vi "RFSG List Mode Test Signal Generation for 5668 with calibrated Signal.vi"(0 "Resource Name":refnum<k15>="RFSG" caption="resource name", 5 "Start Frequency":dbl=3850000000.0 format="%#_6p", 7 "End Frequency":dbl=4800000000.0 format="%#_6p", 11 "error in (no error)":errorcluster) -> (4 "# Tones":i32, 15 "error out":errorcluster)   [LabVIEW 2017]
doc: "Demonstrates how to create a Configuration List for sweeping frequency and/or power."
uses:
  <instrlib>/niRFSG/niRFSG.llb/niRFSG Ref Clock Sources.ctl
  <instrlib>/niRFSG/niRFSG.llb/niRFSG Configuration List Properties.ctl
  <vilib>/Analysis/1siggen.llb/Ramp Pattern by Delta.vi
  <vilib>/Analysis/NI_AALBase.lvlib
panel:
  in  "delta":dbl=50000000.0 format="%#_6p"
  out "Ramp Pattern":dbl[](array[numeric]) format="%#_6p"
  in  "Power Level (dBm)":dbl format="%_3f"
  in  "Timer:Interval":dbl
  in  "List Trigger Source":string(combo)="PXI_Trig1"
  out "Current Frequency (Hz)":dbl format="%#.3p"
  in  "Frequency Settling (ppm)":dbl=1.0 format="%#.6f"
  in  "Stop":bool
  in  "Reference Clock Source":T1="OnboardClock"
  # "Overview: Demonstrates how to create a Configuration List for sweeping frequency and/or power.\nRequirements: NI-RFSG\nInstructions:\n1. Change the Resource Name to your device.\n2. Run the VI.\n3. Click Stop to stop the VI."
  # "You can set the Start Frequency and End Frequency parameters to the same value to keep the Frequency or Power Level constant."
  # "In order to configure new settings, you must stop the example using \nthe Stop button and then run the VI with the new settings."
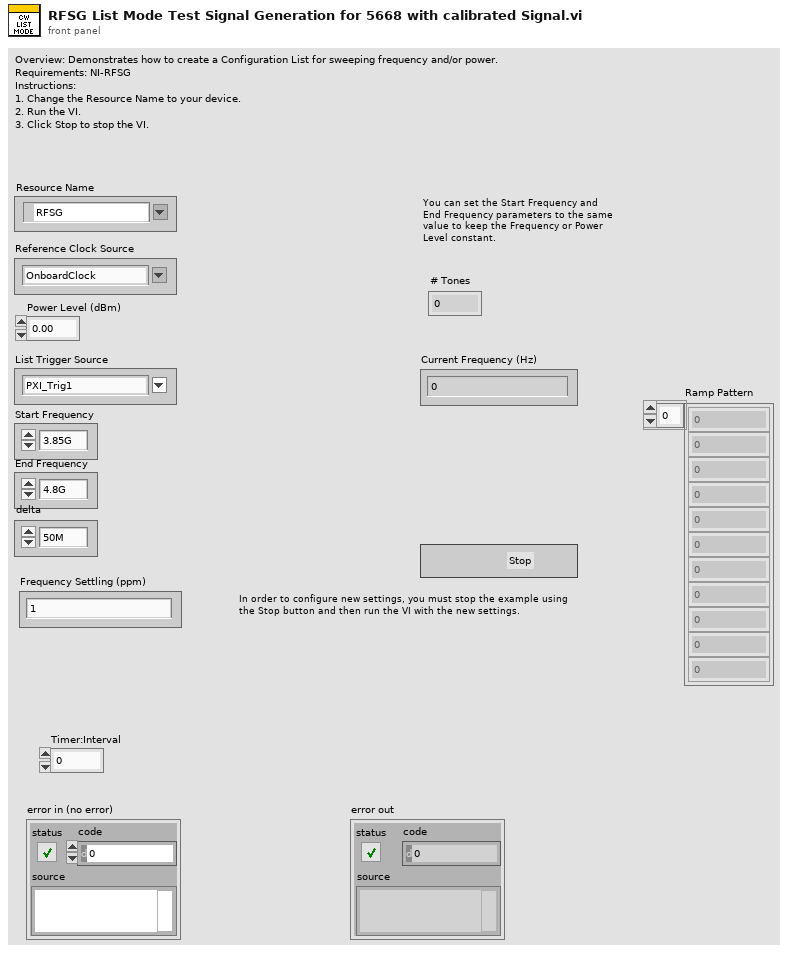
[diagram p1: front panel]
types:
  T1 = typedef "niRFSG Ref Clock Sources.ctl" = string
  T2 = typedef "niRFSG Configuration List Properties.ctl" = u32
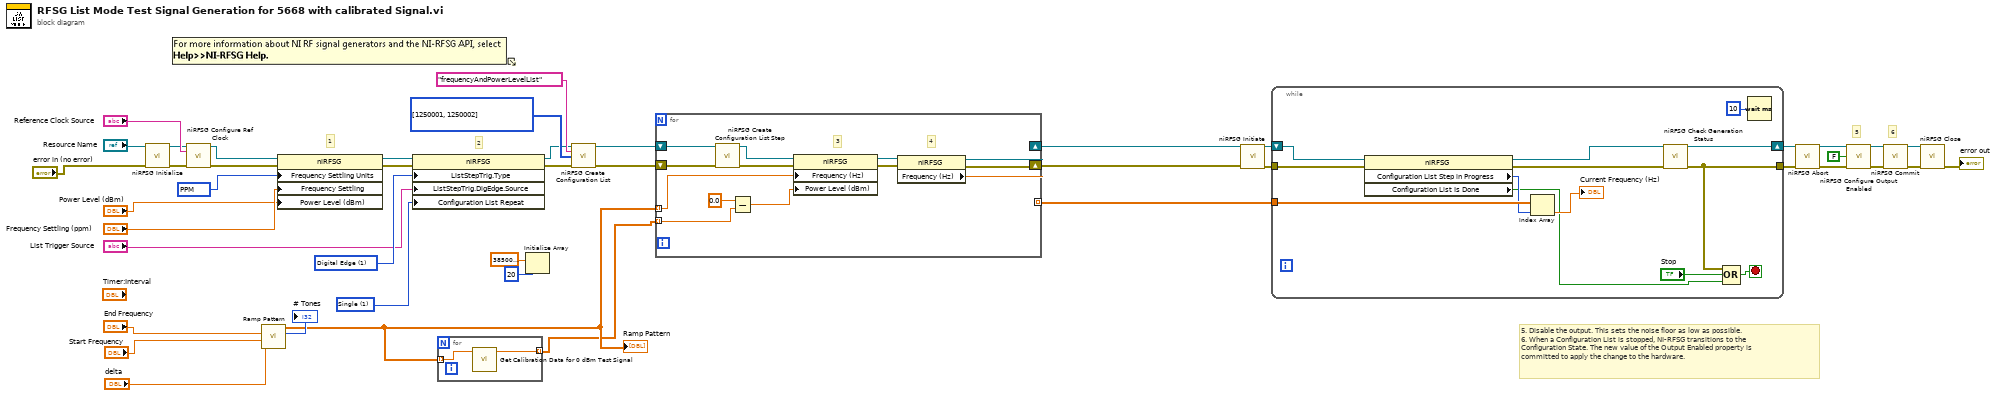
[diagram p0: block diagram]
diagram:
  w9 = 1 items=["Continuous", "Single"] ("Configuration List:Configuration List Repeat")
  w32 = T2[] [1250001, 1250002] items=["ALC Control"=1150195, "Amp Path"=1150185, "Amplitude Settling (dB)"=1150137, "Attenuator Setting (dB)"=1150173, "Automatic Power Search"=1150196, "Frequency (Hz)"=1250001, "Frequency Settling"=1150083, "IQ Out Port Carrier Frequency"=1150145, "IQ Out Port Common Mode Offset"=1150148, "IQ Out Port Level"=1150147, "IQ Out Port Offset"=1150149, "Output Enabled"=1250004, "Phase Offset (Degrees)"=1150024, "Power Level (dBm)"=1250002, "Pulse Modulation Enabled"=1250051, "Timer Event Interval (s)"=1150100, "Upconverter Center Frequency (Hz)"=1154098] ("configuration list properties")
  w39 = 1 items=["None", "Digital Edge", "Software"] ("Triggers:Configuration List Step:Type")
  w44 = 12002 items=["Seconds After Lock"=12000, "Seconds After I/O"=12001, "PPM"=12002] ("RF:Frequency Settling Units")
  # "6"
  # "2"
  # "5. Disable the output. This sets the noise floor as low as possible.\n6. When a Configuration List is stopped, NI-RFSG transitions to the Configuration State. The new value of the Output Enabled property is committed to apply the change to the hardware."
  # "5"
  # "1"
  n1 = call <instrlib>:"niRFSG Initialize.vi"("resource name"="Resource Name", "error in"="error in (no error)") -> ("instrument handle"=w22:refnum<k15>, "error out"=w21:errorcluster)  [unwired: 2 in, 10 out]
  n2 = call <instrlib>:"niRFSG Configure Ref Clock.vi"("instrument handle"=w22, "ref clock source"="Reference Clock Source", "error in"=w21) -> ("instrument handle out"=w11:refnum<k15>, "error out"=w26:errorcluster)  [unwired: 1 in, 10 out]
  n3 = call-poly <vilib>:"Ramp Pattern.vi"("start"="Start Frequency", "end"="End Frequency", "delta"="delta") -> ("samples"=→"# Tones":i32, "Ramp Pattern"=w2:dbl[])  [unwired: 6 in, 1 out]
  "Ramp Pattern" <- w2
  n4 = property class="niRFSG"(reference=w11, error in=w26, "Frequency Settling Units"=w44, "Frequency Settling"="Frequency Settling (ppm)", "Power Level (dBm)"="Power Level (dBm)") -> (reference out=w36:refnum<k15>, error out=w37:errorcluster)
  n5 = property class="niRFSG"(reference=w36, error in=w37, "ListStepTrig.Type"=w39, "ListStepTrig.DigEdge.Source"="List Trigger Source", "Configuration List Repeat"=w9) -> (reference out=w25:refnum<k15>, error out=w33:errorcluster)
  n6 = for {
    tunnel: w2 -> [w46] mode=indexing
    tunnel: [w45] -> w1 mode=indexing
    n7 = call "Get Calibration Data for 0 dBm Test Signal.vi"("Carrier Frequency"=w46) -> ("Calibration Data"=w45:dbl)  [unwired: 9 in, 1 out]
  }
  n8 = Initialize Array(3850000000.0 ("element"), 20 ("dimension size")) -> ()  [unwired: 1 out]
  n9 = call <instrlib>:"niRFSG Create Configuration List.vi"("instrument handle"=w25, "list name"="frequencyAndPowerLevelList", "configuration list properties"=w32, "error in"=w33) -> ("instrument handle out"=w19:refnum<k15>, "error out"=w38:errorcluster)  [unwired: 1 in, 9 out]
  n10 = for {
    shift-right: [w54] -> w15
    shift-left: w19 -> [w52]
    shift-right: [w55] -> w14
    shift-left: w38 -> [w51]
    tunnel: [w56] -> w20 mode=indexing
    tunnel: w2 -> [w50] mode=indexing
    tunnel: w1 -> [w49] mode=indexing
    # "4"
    # "3"
    n11 = call <instrlib>:"niRFSG Create Configuration List Step.vi"("instrument handle"=w52, "error in"=w51) -> ("instrument handle out"=w59:refnum<k15>, "error out"=w53:errorcluster)  [unwired: 1 in, 11 out]
    n12 = Subtract(x=0.0, y=w49) -> (x-y=w47:dbl)
    n13 = property class="niRFSG"(reference=w59, error in=w53, "Frequency (Hz)"=w50, "Power Level (dBm)"=w47) -> (reference out=w58:refnum<k15>, error out=w57:errorcluster)
    n14 = property class="niRFSG"(reference=w58, error in=w57) -> (reference out=w54:refnum<k15>, error out=w55:errorcluster, "Frequency (Hz)"=w56:dbl)
  }
  n15 = call <instrlib>:"niRFSG Initiate.vi"("instrument handle"=w15, "error in"=w14) -> ("instrument handle out"=w42:refnum<k15>, "error out"=w17:errorcluster)  [unwired: 12 out]
  n16 = while {
    shift-right: [w67] -> w40
    shift-left: w42 -> [w66]
    tunnel: w20 -> [w70]
    tunnel: [w65] -> w18
    tunnel: w17 -> [w64]
    stop <- w72 stop-if-true
    n17 = property class="niRFSG"(reference=w66, error in=w64) -> (reference out=w62:refnum<k15>, error out=w63:errorcluster, "Configuration List Step in Progress"=w69:i64, "Configuration List Is Done"=w60:bool)
    n18 = Index Array(array=w70, index=w69) -> (element=→"Current Frequency (Hz)":dbl)
    n19 = call <instrlib>:"niRFSG Check Generation Status.vi"("instrument handle"=w62, "error in"=w63) -> ("instrument handle out"=w67:refnum<k15>, "error out"=w65:errorcluster)  [unwired: 12 out]
    n20 = Compound Arithmetic op=OR(w65, "Stop", w60) -> (w72:bool)
    n21 = Wait (ms)(milliseconds to wait=u32 10) -> ()  [unwired: 1 out]
  }
  n22 = call <instrlib>:"niRFSG Abort.vi"("instrument handle"=w40, "error in"=w18) -> ("instrument handle out"=w24:refnum<k15>, "error out"=w23:errorcluster)  [unwired: 12 out]
  n23 = call <instrlib>:"niRFSG Configure Output Enabled.vi"("instrument handle"=w24, "output enabled"=FALSE ("output enable"), "error in"=w23) -> ("instrument handle out"=w30:refnum<k15>, "error out"=w29:errorcluster)  [unwired: 11 out]
  n24 = call <instrlib>:"niRFSG Commit.vi"("instrument handle"=w30, "error in"=w29) -> ("instrument handle out"=w27:refnum<k15>, "error out"=w28:errorcluster)  [unwired: 12 out]
  n25 = call <instrlib>:"niRFSG Close.vi"("instrument handle"=w27, "error in"=w28) -> ("error out"=→"error out":errorcluster)  [unwired: 13 out]
